vi "Configure Level (Normal).vi"(0 "VISA resource name":refnum<visa-resource-name>, 1 "Auto Mechanical Attenuation (T: Enable)":bool=TRUE, 2 "Mechanical Attenuation Step (0: 2 dB)":i32(ring) items=["2", "10"], 3 "Manual Mechanical Attenuation (10 dB)":dbl=10.0, 5 "Reference Level (0 dBm)":dbl, 7 "Reference Level Offset (0 dB)":dbl, 9 "Amplitude Units (0: dBm)":i32(ring) items=["dBm", "dBmV", "dBmA", "W", "V", "A", "dBuV", "dBuA"], 11 "error in (no error)":errorcluster) -> (4 "VISA resource name out":refnum<visa-resource-name>, 15 "error out":errorcluster)   [LabVIEW 2018, in "Agilent MXA Series.lvlib"]
doc: "Configures the vertical settings of the spectrum analyzer without Electrical Attenuation."
uses:
  Agilent MXA Series.lvlib
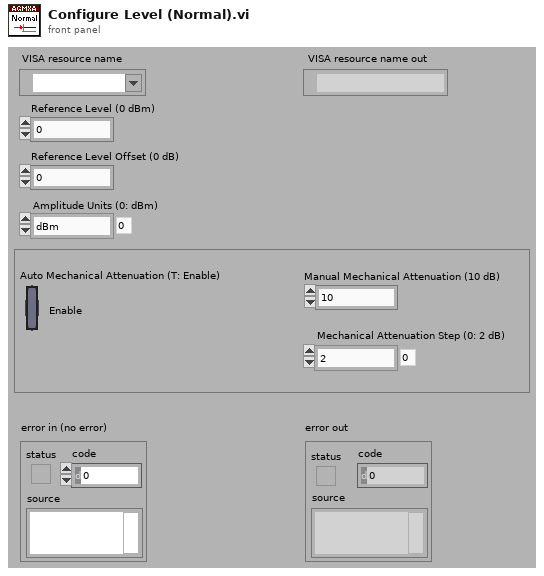
[diagram p1: front panel]
types:
  T1 = typedef "Agilent MXA Series.lvlib/Extended User Data.ctl" = cluster{"Measurement Type":i32, "Agilent MXA/EXA Model":i32}
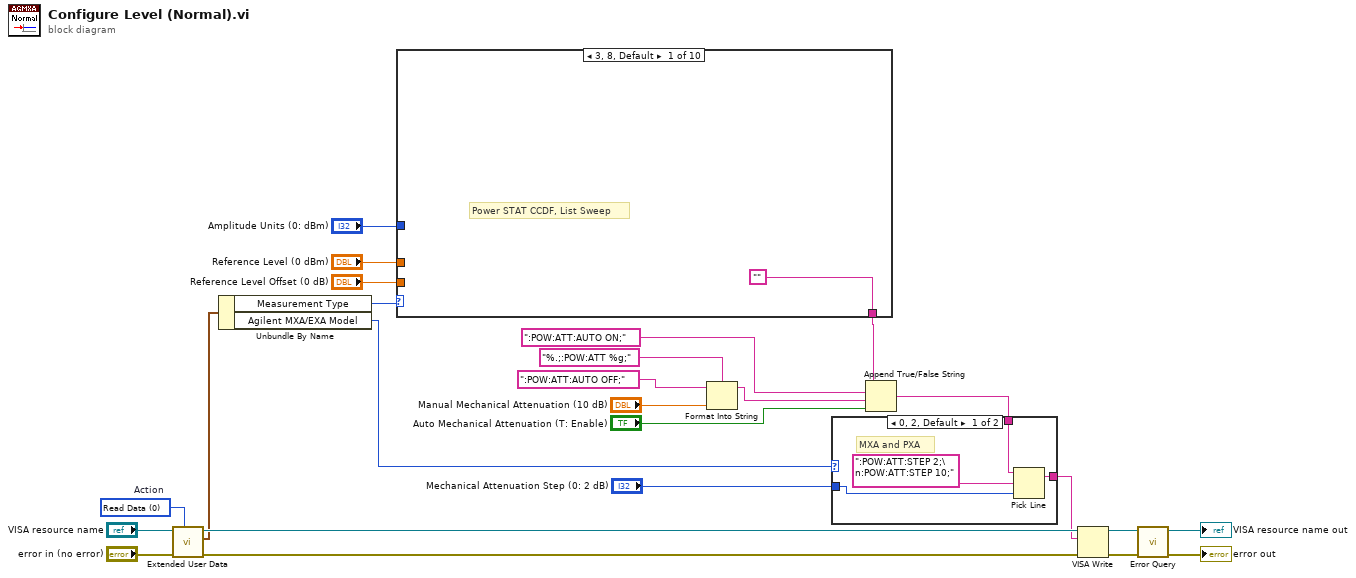
[diagram p0: block diagram]
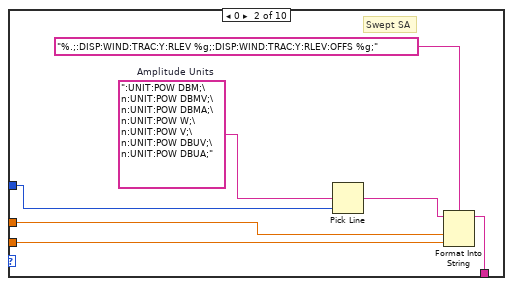
[diagram p3: hidden frame]
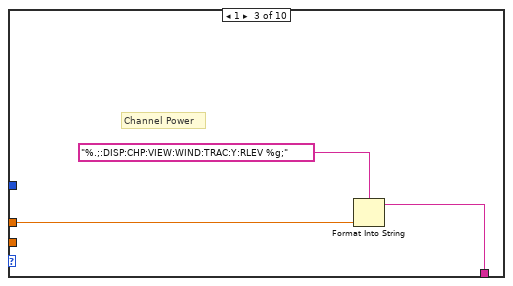
[diagram p4: hidden frame]
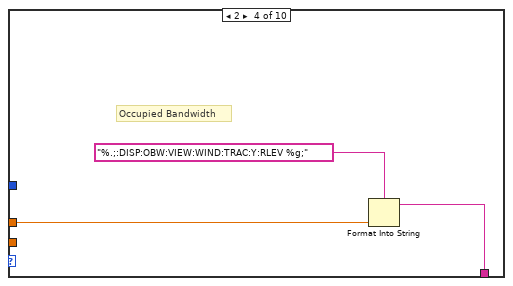
[diagram p5: hidden frame]
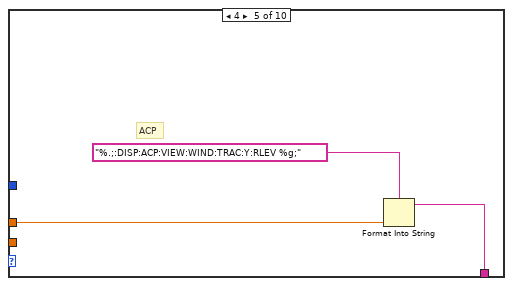
[diagram p6: hidden frame]
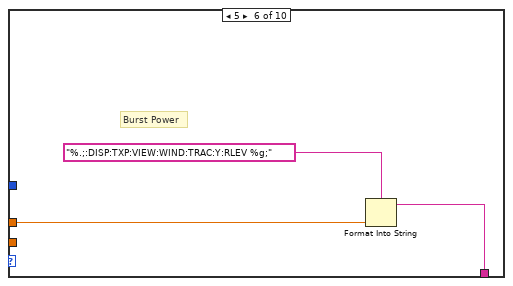
[diagram p7: hidden frame]
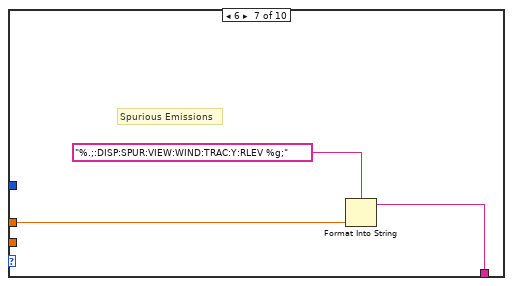
[diagram p8: hidden frame]
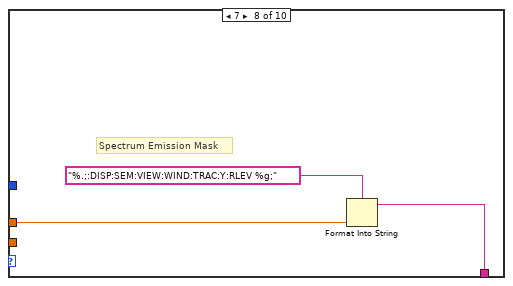
[diagram p9: hidden frame]
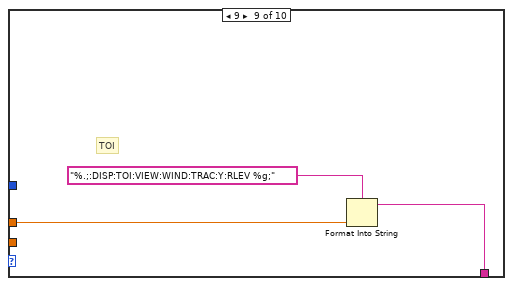
[diagram p10: hidden frame]
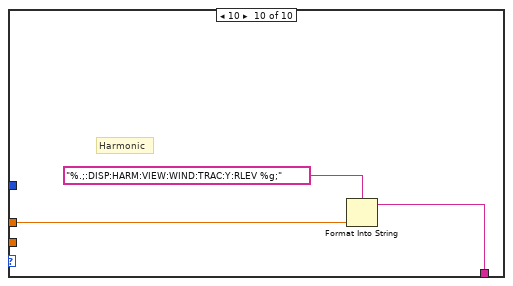
[diagram p11: hidden frame]
diagram:
  w9 = 0 items=["Read Data", "Write Data", "Clear Data", "Clear ALL Data"]  # Action
  n1 = call "Extended User Data.vi"("Action (1:Write Data)"=w9, "Error In (no error)"="error in (no error)", "VISA resource name in"="VISA resource name") -> ("Error Out"=w18:errorcluster, "User Data Out"=w14:T1, "VISA resource name out"=w19:refnum<visa-resource-name>)  [unwired: 6 in]
  n2 = Unbundle By Name(w14) -> ("Measurement Type"=w13:i32, "Agilent MXA/EXA Model"=w3:i32)
  n3 = case shown="3, 8, Default" w13 {
    tunnel: "Reference Level (0 dBm)" -> [_ w29 w35 w38 w41 w44 w47 w50 w53 w56]
    tunnel: "Reference Level Offset (0 dB)" -> [_ w28 _ _ _ _ _ _ _ _]
    tunnel: "Amplitude Units (0: dBm)" -> [_ w30 _ _ _ _ _ _ _ _]
    tunnel: ["" w27 w34 w37 w40 w43 w46 w49 w52 w55] -> w5
    frame 3, 8, Default {
      # "Power STAT CCDF, List Sweep"
    }
    frame 0 {
      w32 = ":UNIT:POW DBM;\n:UNIT:POW DBMV;\n:UNIT:POW DBMA;\n:UNIT:POW W;\n:UNIT:POW V;\n:UNIT:POW DBUV;\n:UNIT:POW DBUA;"  # Amplitude Units
      # "Swept SA"
      n4 = Pick Line(multi-line string=w32, line index=w30) -> (output string=w31:string)  [unwired: 1 in]
      n5 = Format Into String(format string="%.;:DISP:WIND:TRAC:Y:RLEV %g;:DISP:WIND:TRAC:Y:RLEV:OFFS %g;", initial string=w31, w29, w28) -> (resulting string=w27:string)  [unwired: 1 in, 1 out]
    }
    frame 1 {
      # "Channel Power"
      n6 = Format Into String(format string="%.;:DISP:CHP:VIEW:WIND:TRAC:Y:RLEV %g;", w35) -> (resulting string=w34:string)  [unwired: 2 in, 1 out]
    }
    frame 2 {
      # "Occupied Bandwidth"
      n7 = Format Into String(format string="%.;:DISP:OBW:VIEW:WIND:TRAC:Y:RLEV %g;", w38) -> (resulting string=w37:string)  [unwired: 2 in, 1 out]
    }
    frame 4 {
      # "ACP"
      n8 = Format Into String(format string="%.;:DISP:ACP:VIEW:WIND:TRAC:Y:RLEV %g;", w41) -> (resulting string=w40:string)  [unwired: 2 in, 1 out]
    }
    frame 5 {
      # "Burst Power"
      n9 = Format Into String(format string="%.;:DISP:TXP:VIEW:WIND:TRAC:Y:RLEV %g;", w44) -> (resulting string=w43:string)  [unwired: 2 in, 1 out]
    }
    frame 6 {
      # "Spurious Emissions"
      n10 = Format Into String(format string="%.;:DISP:SPUR:VIEW:WIND:TRAC:Y:RLEV %g;", w47) -> (resulting string=w46:string)  [unwired: 2 in, 1 out]
    }
    frame 7 {
      # "Spectrum Emission Mask"
      n11 = Format Into String(format string="%.;:DISP:SEM:VIEW:WIND:TRAC:Y:RLEV %g;", w50) -> (resulting string=w49:string)  [unwired: 2 in, 1 out]
    }
    frame 9 {
      # "TOI"
      n12 = Format Into String(format string="%.;:DISP:TOI:VIEW:WIND:TRAC:Y:RLEV %g;", w53) -> (resulting string=w52:string)  [unwired: 2 in, 1 out]
    }
    frame 10 {
      # "Harmonic"
      n13 = Format Into String(format string="%.;:DISP:HARM:VIEW:WIND:TRAC:Y:RLEV %g;", w56) -> (resulting string=w55:string)  [unwired: 2 in, 1 out]
    }
  }
  n14 = Format Into String(format string="%.;:POW:ATT %g;", initial string=":POW:ATT:AUTO OFF;", "Manual Mechanical Attenuation (10 dB)") -> (resulting string=w8:string)  [unwired: 1 in, 1 out]
  n15 = Append True/False String(1:"Auto Mechanical Attenuation (T: Enable)", 2:w8, 3:":POW:ATT:AUTO ON;" ("true string"), 4:w5) -> (0:w4:string)
  n16 = case shown="0, 2, Default" w3 {
    tunnel: w4 -> [w60 w62]
    tunnel: [w59 w62] -> w1
    tunnel: "Mechanical Attenuation Step (0: 2 dB)" -> [w58 _]
    frame 0, 2, Default {
      # "MXA and PXA"
      n17 = Pick Line(string ("")=w60, multi-line string=":POW:ATT:STEP 2;\n:POW:ATT:STEP 10;" ("Mechanical Attenuation Step"), line index=w58) -> (output string=w59:string)
    }
    frame 1, 3 {
      # "EXA and CXA"
      # "This command requires installed FSA option and license."
    }
  }
  n18 = VISA Write(VISA resource name=w19, write buffer=w1, error in (no error)=w18) -> (VISA resource name out=w25:refnum<visa-resource-name>, error out=w23:errorcluster)  [unwired: 1 out]
  n19 = call "Error Query.vi"("error in (no error)"=w23, "VISA resource name"=w25) -> ("error out"=→"error out":errorcluster, "VISA resource name out"=→"VISA resource name out":refnum<visa-resource-name>)  [unwired: 6 in, 2 out]
